vi "AutoNamerConfig.vi"(2 "ExtraString":string, 3 "Custom User Path":T1) -> (0 "String":string, 1 "Path":path)   [LabVIEW 2014]
uses:
  Users/mbcsslp2/Control 1.ctl
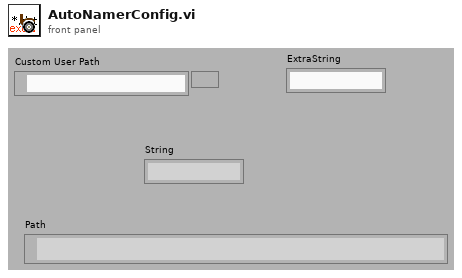
[diagram p1: front panel]
types:
  T1 = typedef "Control 1.ctl" = path
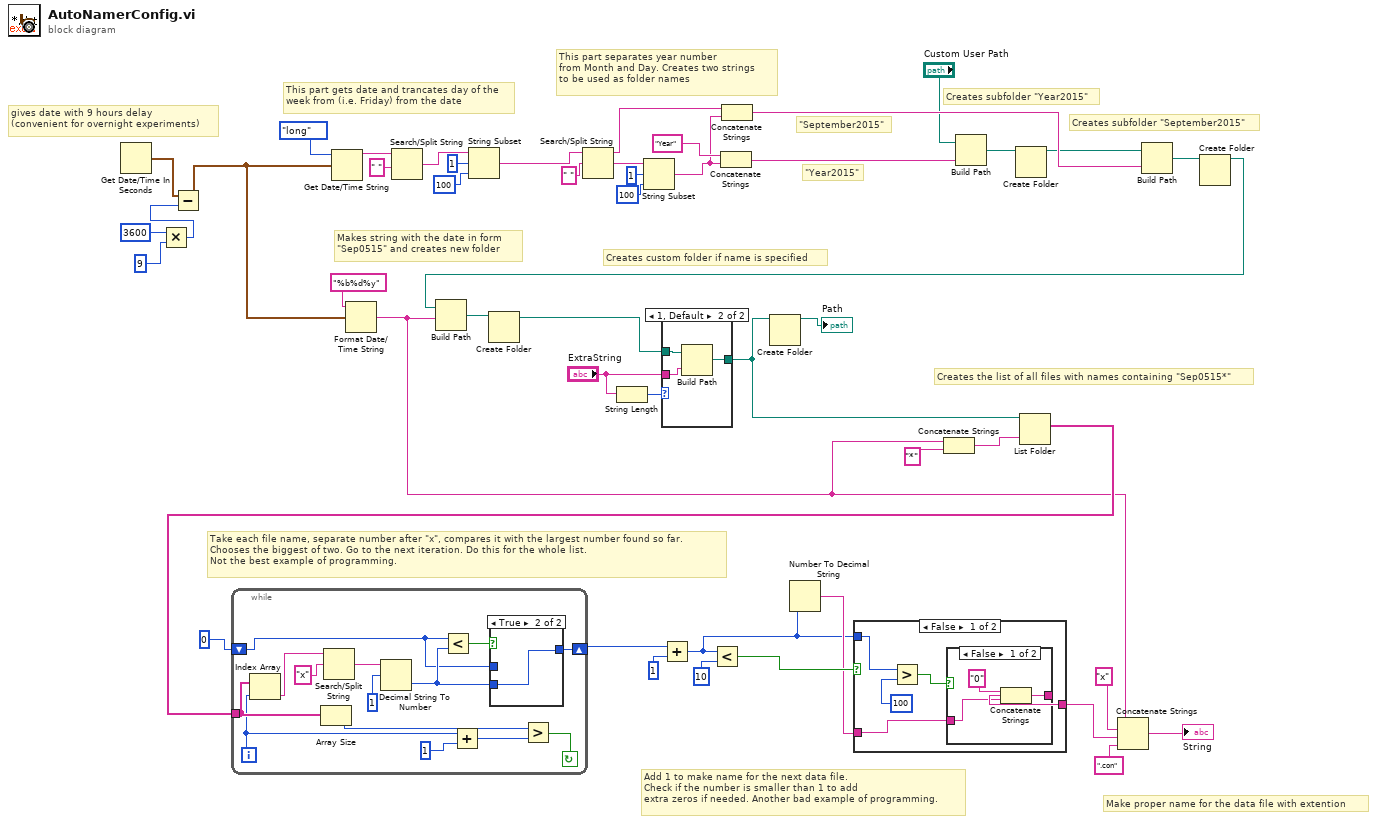
[diagram p0: block diagram]
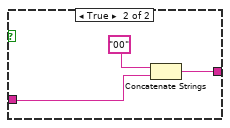
[diagram p5: hidden frame]
diagram:
  # "Make proper name for the data file with extention"
  # "Add 1 to make name for the next data file.\nCheck if the number is smaller than 1 to add\nextra zeros if needed. Another bad example of programming."
  # "Take each file name, separate number after \"x\", compares it with the largest number found so far. \nChooses the biggest of two. Go to the next iteration. Do this for the whole list. \nNot the best example of programming."
  # "Creates the list of all files with names containing \"Sep0515*\""
  # "Creates custom folder if name is specified"
  # "Makes string with the date in form \n\"Sep0515\" and creates new folder"
  # "Creates subfolder \"September2015\""
  # "Creates subfolder \"Year2015\""
  # "\"September2015\""
  # "\"Year2015\""
  # "This part separates year number \nfrom Month and Day. Creates two strings\nto be used as folder names"
  # "This part gets date and trancates day of the\nweek from (i.e. Friday) from the date"
  # "gives date with 9 hours delay\n(convenient for overnight experiments)"
  n1 = Get Date/Time In Seconds() -> (seconds since 1Jan1904=w7:timestamp)
  n2 = Multiply(x=3600, y=9) -> (x*y=w4:i32)
  n3 = Subtract(x=w7, y=w4) -> (x-y=w1:timestamp)
  n4 = Get Date/Time String(date format (0)=enum16{"short", "long", "abbreviated"}."long", seconds (now)=w1) -> (date string=w34:string)  [unwired: 1 in, 1 out]
  n5 = Format Date/Time String(time format string (%c)="%b%d%y", seconds (now)=w1) -> (date/time string=w19:string)  [unwired: 1 in]
  n6 = Search/Split String(string=w34, search string/char (-)=" ") -> (match + rest of string=w32:string)  [unwired: 1 in, 2 out]
  n7 = String Subset(string=w32, offset (0)=1, length (rest)=100 ("length (rest)")) -> (substring=w25:string)
  n8 = Search/Split String(string=w25, search string/char (-)=" ") -> (substring before match=w21:string, match + rest of string=w26:string)  [unwired: 1 in, 1 out]
  n9 = String Length(string="ExtraString") -> (length=w3:i32)
  n10 = String Subset(string=w26, offset (0)=1, length (rest)=100 ("length (rest)")) -> (substring=w22:string)
  n11 = Concatenate Strings("Year" ("Substring"), w22) -> (w23:string)
  n12 = Concatenate Strings(w21, w22) -> (w20:string)
  n13 = Concatenate Strings(w19, "*") -> (w42:string)
  n14 = Build Path(base path="Custom User Path", name or relative path=w23) -> (appended path=w18:path)
  n15 = Create Folder(path (use dialog)=w18) -> (created path=w17:path)  [unwired: 2 in, 2 out]
  n16 = Build Path(base path=w17, name or relative path=w20) -> (appended path=w16:path)
  n17 = Create Folder(path (use dialog)=w16) -> (created path=w15:path)  [unwired: 2 in, 2 out]
  n18 = Build Path(base path=w15, name or relative path=w19) -> (appended path=w8:path)
  n19 = Create Folder(path (use dialog)=w8) -> (created path=w9:path)  [unwired: 2 in, 2 out]
  n20 = case shown="1, Default" w3 {
    tunnel: [w49 w52] -> w10
    tunnel: w9 -> [w49 w51]
    tunnel: "ExtraString" -> [_ w50]
    frame 0 {
    }
    frame 1, Default {
      n21 = Build Path(base path=w51, name or relative path=w50) -> (appended path=w52:path)
    }
  }
  n22 = Create Folder(path (use dialog)=w10) -> (created path=→"Path":path)  [unwired: 2 in, 2 out]
  n23 = List Folder(path=w10, pattern=w42) -> (filenames=w43:string[])  [unwired: 2 in, 3 out]
  n24 = while {
    shift-left: 0 -> [w59]
    shift-right: [w58] -> w45
    tunnel: w43 -> [w55]
    i -> [w54]
    stop <- w64 continue-if-true
    n25 = Index Array(array=w55, index=w54) -> (element=w63:string)
    n26 = Array Size(array=w55) -> (size(s)=w66:i32)
    n27 = Search/Split String(string=w63, search string/char (-)="x") -> (match + rest of string=w57:string)  [unwired: 1 in, 2 out]
    n28 = Decimal String To Number(string=w57, offset=1) -> (number=w60:i32)  [unwired: 1 in, 1 out]
    n29 = Less?(x=w59, y=w60) -> (x < y?=w61:bool)
    n30 = Add(x=w54, y=1) -> (x+y=w53:i32)
    n31 = case shown="True" w61 {
      tunnel: w60 -> [_ w68]
      tunnel: w59 -> [w67 _]
      tunnel: [w67 w68] -> w58
      frame False {
      }
      frame True {
      }
    }
    n32 = Greater?(x=w66, y=w53) -> (0:w64:bool)
  }
  n33 = Add(x=w45, y=1) -> (x+y=w37:i32)
  n34 = Less?(x=w37, y=10) -> (x < y?=w39:bool)
  n35 = Number To Decimal String(number=w37) -> (decimal integer string=w38:string)  [unwired: 1 in]
  n36 = case shown="False" w39 {
    tunnel: w38 -> [w70 w80]
    tunnel: [w69 w78] -> w36
    tunnel: w37 -> [w72 _]
    frame False {
      n37 = Greater?(x=w72, y=100) -> (0:w71:bool)
      n38 = case shown="False" w71 {
        tunnel: w70 -> [w75 w77]
        tunnel: [w74 w77] -> w69
        frame False {
          n39 = Concatenate Strings("0", w75) -> (w74:string)
        }
        frame True {
        }
      }
    }
    frame True {
      n40 = Concatenate Strings("00", w80) -> (w78:string)
    }
  }
  n41 = Concatenate Strings(w19, "x", w36, ".con" ("Substring")) -> (→"String":string)
